vi "Read Void.vi"(8 "error in":errorcluster, 11 "CoreOOB_Tx in":refnum<class "CIFCoreOOB_Tx.lvclass">) -> (0 "error out":errorcluster, 2 "void":bool, 3 "CoreOOB_Tx out":refnum<class "CIFCoreOOB_Tx.lvclass">)   [LabVIEW 2021, in "CIFCoreOOB_Tx.lvclass"]
uses:
  CIFCoreOOB_Tx.lvclass
  C:/Program Files/National Instruments/LabVIEW 2021/vi.lib/CIF Foundation/CIF Out of Band Commands/CIFOutOfBand.lvclass
  <vilib>/CIF Foundation/CIF Out of Band Commands/CIFOutOfBand.lvclass/CIFOutOfBand.ctl
  <vilib>/CIF Foundation/CIF Out of Band Commands/Accessors/Read Local OOB Data.vi
  CIFCoreOOB_Tx.lvclass/CIFCoreOOB_Tx.ctl
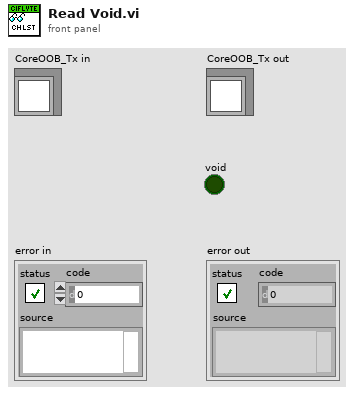
[diagram p1: front panel]
types:
  T1 = typedef "CIFCoreOOB_Tx.lvclass/Template Payload.ctl" = cluster{"void":bool}
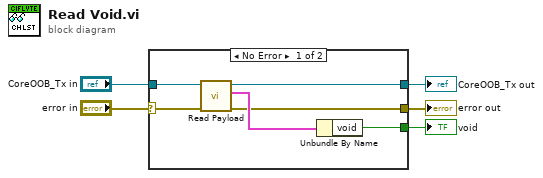
[diagram p0: block diagram]
diagram:
  n1 = case shown="No Error" "error in" {
    selector: "error in" -> [w7 w12]
    tunnel: [w6 w12] -> w4
    tunnel: [w10 w13] -> w2
    tunnel: "CoreOOB_Tx in" -> [w11 w13]
    tunnel: [w8 _] -> w1
    frame No Error {
      n2 = call "Read Payload.vi"("error in"=w7, "CoreOOB_Tx in"=w11) -> ("error out"=w6:errorcluster, "data"=w9:T1, "CoreOOB_Tx out"=w10:refnum<class "CIFCoreOOB_Tx.lvclass">)  [unwired: 7 in]
      n3 = Unbundle By Name(w9) -> ("void"=w8:bool)
    }
    frame Error {
    }
  }
  "error out" <- w4
  "CoreOOB_Tx out" <- w2
  "void" <- w1
